vi "Ej_6_Queue.vi"() -> ()   [LabVIEW 2021]
panel:
  out "Numeric":dbl
  out "Waveform Chart":dbl(graph)
  in  "stop":bool
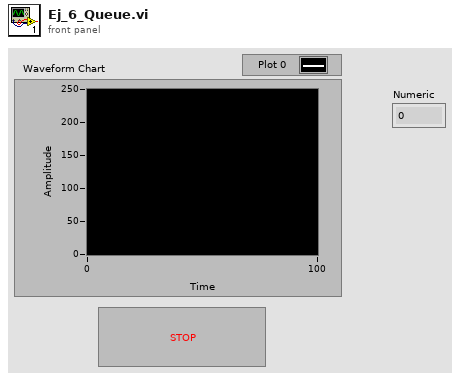
[diagram p1: front panel]
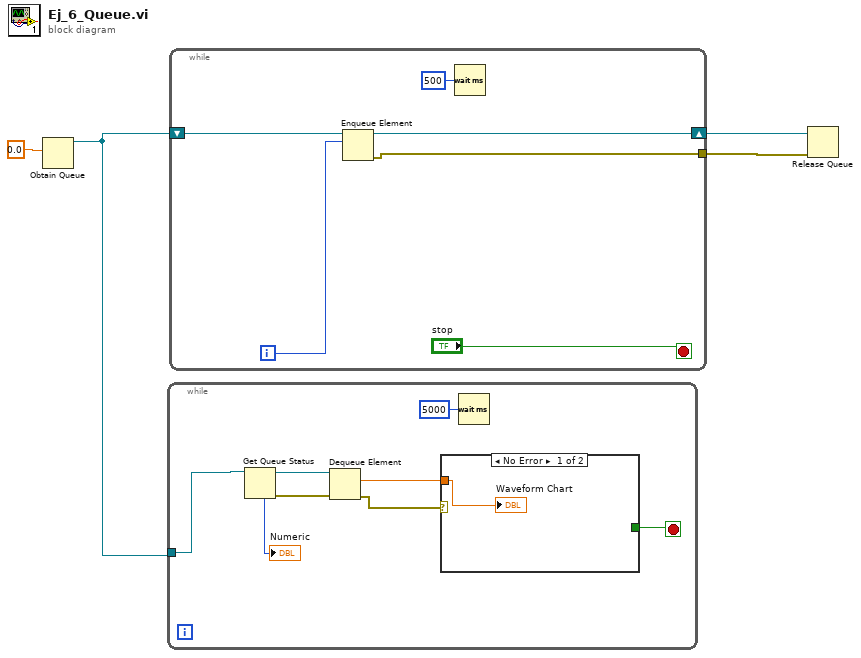
[diagram p0: block diagram]
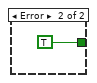
[diagram p2: hidden frame]
diagram:
  n1 = Obtain Queue(element data type=0.0) -> (queue out=w3:refnum<queue>)  [unwired: 4 in, 2 out]
  n2 = while {
    tunnel: w3 -> [w8]
    stop <- w9 stop-if-true
    n3 = Get Queue Status(queue=w8) -> (queue out=w7:refnum<queue>, error out=w5:errorcluster, # elements in queue=→"Numeric":i32)  [unwired: 2 in, 5 out]
    n4 = Dequeue Element(queue=w7, error in (no error)=w5) -> (element=w10:dbl, error out=w11:errorcluster)  [unwired: 1 in, 2 out]
    n5 = case shown="No Error" w11 {
      tunnel: w10 -> [w13 _]
      tunnel: [_ TRUE] -> w9
      frame No Error {
        "Waveform Chart" <- w13
      }
      frame Error {
      }
    }
    n6 = Wait (ms)(milliseconds to wait=u32 5000) -> ()  [unwired: 1 out]
  }
  n7 = while {
    shift-right: [w19] -> w2
    shift-left: w3 -> [w20]
    tunnel: [w16] -> w1
    i -> [w18]
    stop <- "stop" stop-if-true
    n8 = Enqueue Element(queue=w20, element=w18) -> (queue out=w19:refnum<queue>, error out=w16:errorcluster)  [unwired: 2 in, 1 out]
    n9 = Wait (ms)(milliseconds to wait=u32 500) -> ()  [unwired: 1 out]
  }
  n10 = Release Queue(queue=w2, error in (no error)=w1) -> ()  [unwired: 1 in, 3 out]
